vi "Vision Processing.vi"(4 "error in (no error)":errorcluster, 7 "Image Size":T1=enum."320x240") -> ()   [LabVIEW 2017]
doc: "This VI runs in parallel to other tasks. It gets images from the camera, processes them for color or shape and use that information to affect robot behavior."
uses:
  <vilib>/Rock Robotics/WPI/Camera/WPI_CameraImageSize.ctl
  <vilib>/Rock Robotics/WPI/Camera/WPI_CameraWhite Balance Values.ctl
  <vilib>/Rock Robotics/WPI/Camera/WPI_CameraExposure Values.ctl
  <vilib>/Rock Robotics/WPI/Camera/WPI_CameraFrameRate.ctl
  Robot Global Data.vi
panel:
  in  "Image Size 2":T1=enum."320x240"
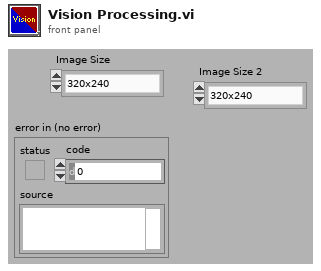
[diagram p1: front panel]
types:
  T1 = typedef "WPI_CameraImageSize.ctl" = enum16{"640x480", "320x240", "160x120", "Custom"}
  T2 = typedef "WPI_CameraFrameRate.ctl" = u32
  T3 = typedef "WPI_CameraExposure Values.ctl" = enum16{"Auto", "Flicker-free 50 Hz", "Flicker-free 60 Hz", "Hold current", "Custom"}
  T4 = typedef "WPI_CameraWhite Balance Values.ctl" = enum16{"Auto", "Fixed indoor", "Fixed outdoor 1", "Fixed outdoor 2", "Fixed fluorescent 1", "Fixed fluorescent 2", "Hold current", "Custom"}
  T5 = typedef "Image Type" = u32
  T6 = typedef "WPI_CameraDevRef.ctl" = cluster{"Camera Address":string, "CameraStatus":errorcluster}
  T7 = typedef "IMAQ Image.ctl" = refnum<image>
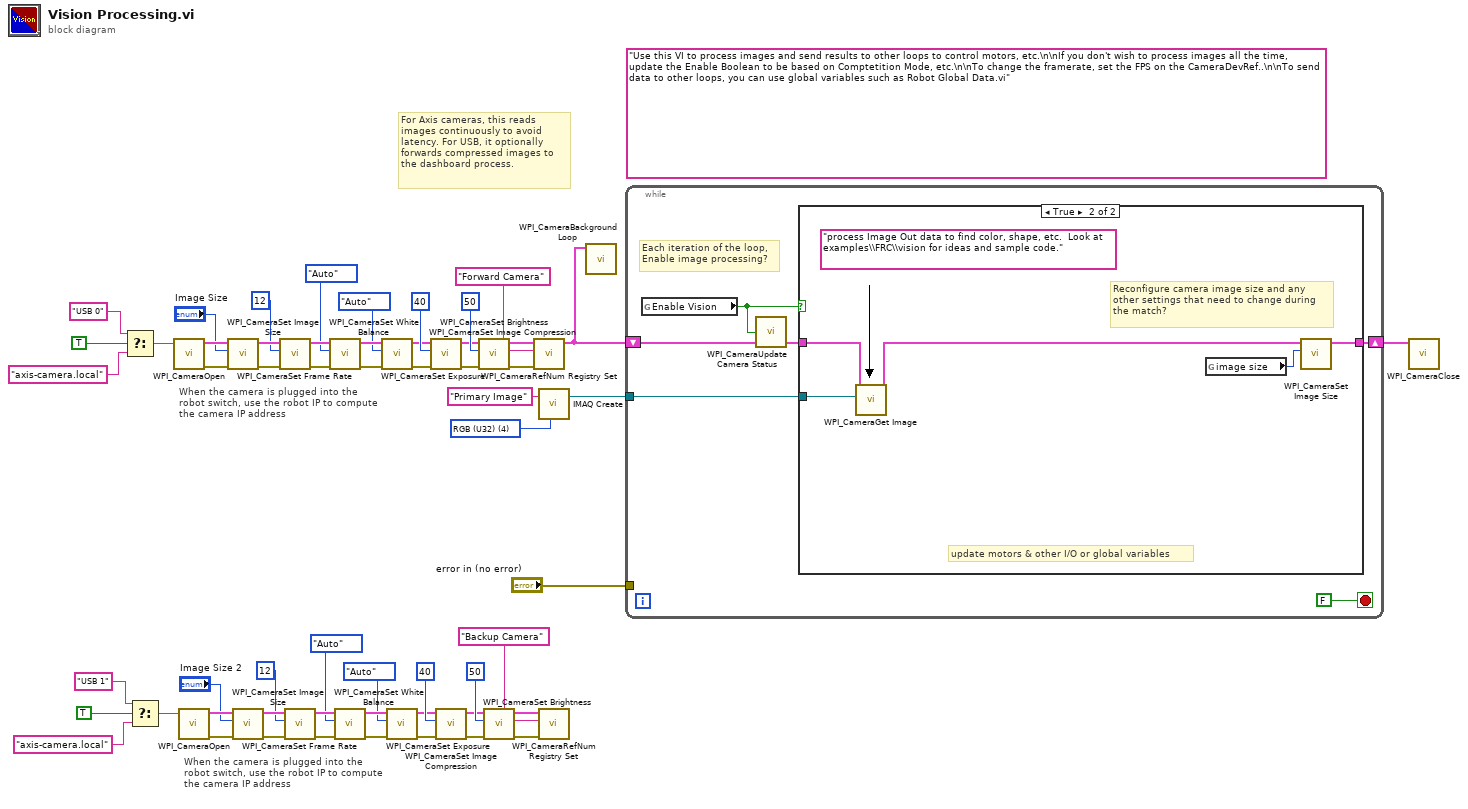
[diagram p0: block diagram]
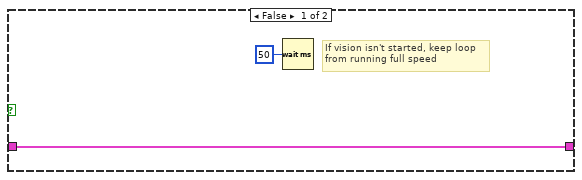
[diagram p2: hidden frame]
diagram:
  (unwired) "Use this VI to process images and send results to other loops to control motors, etc.\n\nIf you don't wish to process images all the time, update the Enable Boolean to be based on Comptetition Mode, etc.\n\nTo change the framerate, set the FPS on the CameraDevRef..\n\nTo send data to other loops, you can use global variables such as Robot Global Data.vi"
  w56 = T5 4 items=["Grayscale (U8)", "Grayscale (I16)", "Grayscale (SGL)", "Complex (CSG)", "RGB (U32)", "HSL (U32)", "RGB (U64)"] ("Image Type")
  # "When the camera is plugged into the\nrobot switch, use the robot IP to compute\nthe camera IP address"
  # "When the camera is plugged into the\nrobot switch, use the robot IP to compute\nthe camera IP address"
  # "For Axis cameras, this reads\nimages continuously to avoid\nlatency. For USB, it optionally\nforwards compressed images to\nthe dashboard process."
  n1 = Select(t="USB 0" ("format string"), s=TRUE ("dot notation? (F)"), f="axis-camera.local" ("format string")) -> (s? t:f=w27:string)
  n2 = Select(t="USB 1" ("format string"), s=TRUE ("dot notation? (F)"), f="axis-camera.local" ("format string")) -> (s? t:f=w2:string)
  n3 = call <vilib>:"WPI_CameraOpen.vi"("Camera Address"=w27) -> ("error out"=w44:errorcluster, "CameraDevRef"=w45:T6)  [unwired: 2 in, 7 out]
  n4 = call <vilib>:"WPI_CameraOpen.vi"("Camera Address"=w2) -> ("error out"=w16:errorcluster, "CameraDevRef"=w17:T6)  [unwired: 2 in, 7 out]
  n5 = call <vilib>:"WPI_CameraSet Image Size.vi"("error in (no error)"=w44, "Image Size"="Image Size", "CameraDevRef"=w45) -> ("error out"=w43:errorcluster, "CameraDevRef Out"=w46:T6)  [unwired: 1 in, 6 out]
  n6 = call <vilib>:"WPI_CameraSet Image Size.vi"("error in (no error)"=w16, "Image Size"="Image Size 2", "CameraDevRef"=w17) -> ("error out"=w15:errorcluster, "CameraDevRef Out"=w18:T6)  [unwired: 1 in, 6 out]
  n7 = call <vilib>:"WPI_CameraSet Frame Rate.vi"("error in (no error)"=w43, "Frame Rate (fps)"=T2 12, "CameraDevRef"=w46) -> ("error out"=w42:errorcluster, "CameraDevRef Out"=w48:T6)  [unwired: 7 out]
  n8 = call <vilib>:"WPI_CameraSet Frame Rate.vi"("error in (no error)"=w15, "Frame Rate (fps)"=T2 12, "CameraDevRef"=w18) -> ("error out"=w14:errorcluster, "CameraDevRef Out"=w20:T6)  [unwired: 7 out]
  n9 = call <vilib>:"WPI_CameraSet White Balance.vi"("error in (no error)"=w42, "White Balance"=WPI_CameraWhite_Balance_Values."Auto", "CameraDevRef"=w48) -> ("error out"=w41:errorcluster, "CameraDevRef Out"=w47:T6)  [unwired: 1 in, 6 out]
  n10 = call <vilib>:"WPI_CameraSet White Balance.vi"("error in (no error)"=w14, "White Balance"=WPI_CameraWhite_Balance_Values."Auto", "CameraDevRef"=w20) -> ("error out"=w13:errorcluster, "CameraDevRef Out"=w19:T6)  [unwired: 1 in, 6 out]
  n11 = call <vilib>:"WPI_CameraSet Exposure.vi"("error in (no error)"=w41, "Exposure"=WPI_CameraExposure_Values."Auto", "CameraDevRef"=w47) -> ("error out"=w40:errorcluster, "CameraDevRef Out"=w50:T6)  [unwired: 1 in, 6 out]
  n12 = call <vilib>:"WPI_CameraSet Exposure.vi"("error in (no error)"=w13, "Exposure"=WPI_CameraExposure_Values."Auto", "CameraDevRef"=w19) -> ("error out"=w12:errorcluster, "CameraDevRef Out"=w22:T6)  [unwired: 1 in, 6 out]
  n13 = call <vilib>:"WPI_CameraSet Image Compression.vi"("error in (no error)"=w40, "Compression"=40, "CameraDevRef"=w50) -> ("error out"=w39:errorcluster, "CameraDevRef Out"=w49:T6)  [unwired: 7 out]
  n14 = call <vilib>:"WPI_CameraSet Image Compression.vi"("error in (no error)"=w12, "Compression"=40, "CameraDevRef"=w22) -> ("error out"=w11:errorcluster, "CameraDevRef Out"=w21:T6)  [unwired: 7 out]
  n15 = call <vilib>:"WPI_CameraSet Brightness.vi"("error in (no error)"=w39, "Brightness"=50, "CameraDevRef"=w49) -> ("error out"=w37:errorcluster, "CameraDevRef Out"=w38:T6)  [unwired: 1 in, 6 out]
  n16 = call <vilib>:"WPI_CameraSet Brightness.vi"("error in (no error)"=w11, "Brightness"=50, "CameraDevRef"=w21) -> ("error out"=w9:errorcluster, "CameraDevRef Out"=w10:T6)  [unwired: 1 in, 6 out]
  n17 = call <vilib>:"WPI_CameraRefNum Registry Set.vi"("error in (no error)"=w37, "refnum name"="Forward Camera", "CameraDevRef"=w38) -> ("CameraDevRef"=w33:T6)  [unwired: 1 in, 7 out]
  n18 = call "IMAQ Create"("Image Name"="Primary Image", "Image Type"=w56) -> ("New Image"=w54:T7)  [unwired: 2 in, 2 out]
  n19 = call <vilib>:"WPI_CameraRefNum Registry Set.vi"("error in (no error)"=w9, "refnum name"="Backup Camera", "CameraDevRef"=w10) -> ()  [unwired: 1 in, 8 out]
  n20 = call <vilib>:"WPI_CameraBackground Loop.vi"("CameraDevRef"=w33) -> ()  [unwired: 11 in]
  n21 = while {
    shift-right: [w61] -> w31
    shift-left: w33 -> [w59]
    tunnel: w54 -> [w60]
    tunnel: "error in (no error)" -> [_]
    stop <- FALSE stop-if-true
    # "Each iteration of the loop,\nEnable image processing?"
    n22 = global read "Robot Global Data.vi" "Enable Vision"() -> (w57:bool)
    n23 = call <vilib>:"WPI_CameraUpdate Camera Status.vi"("CameraDevRef In"=w59, "Enable Vision"=w57) -> ("CameraDevRef Out"=w58:T6)  [unwired: 3 in]
    n24 = case shown="True" w57 {
      tunnel: w60 -> [_ w68]
      tunnel: [w64 w69] -> w61
      tunnel: w58 -> [w64 w66]
      frame False {
        # "If vision isn't started, keep loop\nfrom running full speed"
        n25 = Wait (ms)(milliseconds to wait=u32 50) -> ()  [unwired: 1 out]
      }
      frame True {
        (unwired) "process Image Out data to find color, shape, etc.  Look at examples\\FRC\\vision for ideas and sample code."
        # "update motors & other I/O or global variables"
        # "Reconfigure camera image size and any\nother settings that need to change during\nthe match?"
        n26 = call <vilib>:"WPI_CameraGet Image.vi"("Image"=w68, "CameraDevRef"=w66) -> ("CameraDevRef Out"=w65:T6)  [unwired: 1 in, 8 out]
        n27 = global read "Robot Global Data.vi" "image size"() -> (w67:T1)
        n28 = call <vilib>:"WPI_CameraSet Image Size.vi"("Image Size"=w67, "CameraDevRef"=w65) -> ("CameraDevRef Out"=w69:T6)  [unwired: 2 in, 7 out]
      }
    }
  }
  n29 = call <vilib>:"WPI_CameraClose.vi"("CameraDevRef"=w31) -> ()  [unwired: 1 in, 10 out]
